vi "Get_folder_and_filenames.vi"(0 "file path (dialog if empty)":path) -> (1 "Folders":path[](array[path]), 2 "Files":path[](array[path]))   [LabVIEW 2012]
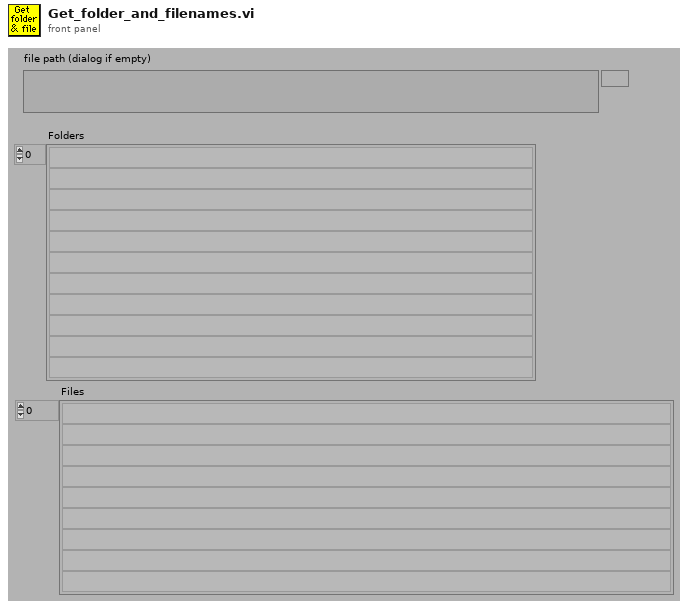
[diagram p1: front panel]
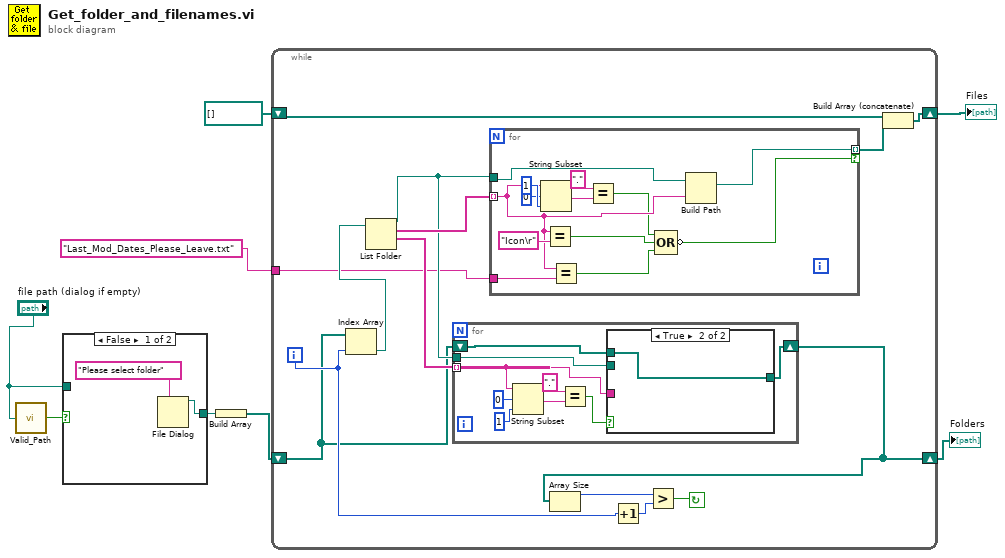
[diagram p0: block diagram]
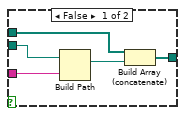
[diagram p2: hidden frame]
diagram:
  n1 = call "Valid_Path.vi"("Filename"="file path (dialog if empty)") -> ("Valid Path?"=w4:bool)
  n2 = case shown="False" w4 {
    tunnel: [w10 w11] -> w7
    tunnel: "file path (dialog if empty)" -> [_ w11]
    frame False {
      n3 = File Dialog(7:"Please select folder" ("prompt")) -> (3:w10:path)  [unwired: 1 in, 8 out]
    }
    frame True {
    }
  }
  n4 = Build Array(w7) -> (w6:path[])
  n5 = while {
    shift-left: w6 -> [w17]
    shift-right: [w16] -> w8
    tunnel: "Last_Mod_Dates_Please_Leave.txt" -> [w15]
    shift-right: [w12] -> w1
    shift-left: path[] [] -> [w14]
    i -> [w23]
    stop <- w22 continue-if-true
    n6 = Index Array(array=w17, index=w23) -> (element=w25:path)
    n7 = List Folder(path=w25) -> (path out=w19:path, filenames=w20:string[], folder names=w18:string[])  [unwired: 1 in, 3 out]
    n8 = for {
      tunnel: w19 -> [w29]
      tunnel: w18 -> [w28] mode=indexing
      shift-right: [w26] -> w16
      shift-left: w17 -> [w27]
      n9 = String Subset(string=w28, offset (0)=0, length (rest)=1 ("length")) -> (substring=w33:string)
      n10 = Equal?(x=".", y=w33) -> (x = y?=w30:bool)
      n11 = case shown="True" w30 {
        tunnel: w28 -> [w39 _]
        tunnel: w29 -> [w38 _]
        tunnel: w27 -> [w37 w40]
        tunnel: [w35 w40] -> w26
        frame False {
          n12 = Build Path(base path=w38, name or relative path=w39) -> (appended path=w36:path)
          n13 = Build Array (concatenate)(w37, w36) -> (w35:path[])
        }
        frame True {
        }
      }
    }
    n14 = for {
      tunnel: w19 -> [w49]
      tunnel: w20 -> [w46] mode=indexing
      tunnel: [w47] -> w13 mode=indexing if=w41
      tunnel: w15 -> [w45]
      n15 = String Subset(string=w46, offset (0)=0, length (rest)=1 ("length")) -> (substring=w51:string)
      n16 = Equal?(x=w46, y="Icon\r") -> (x = y?=w43:bool)
      n17 = Equal?(x=w46, y=w45) -> (x = y?=w42:bool)
      n18 = Equal?(x=".", y=w51) -> (x = y?=w44:bool)
      n19 = Compound Arithmetic op=OR(w44, w43, w42) -> (invert w41:bool)
      n20 = Build Path(base path=w49, name or relative path=w46) -> (appended path=w47:path)
    }
    n21 = Array Size(array=w16) -> (size(s)=w24:i32)
    n22 = Increment(x=w23) -> (x+1=w21:i32)
    n23 = Greater?(x=w24, y=w21) -> (0:w22:bool)
    n24 = Build Array (concatenate)(w14, w13) -> (w12:path[])
  }
  "Folders" <- w8
  "Files" <- w1
